vi "XuLyStringData.vi"(7 "input cluster":T3) -> (0 "error out":errorcluster, 1 "Return State":T1(ring), 2 "output cluster":T2, 3 "OUT COM 2":refnum<visa-resource-name>)   [LabVIEW 2017]
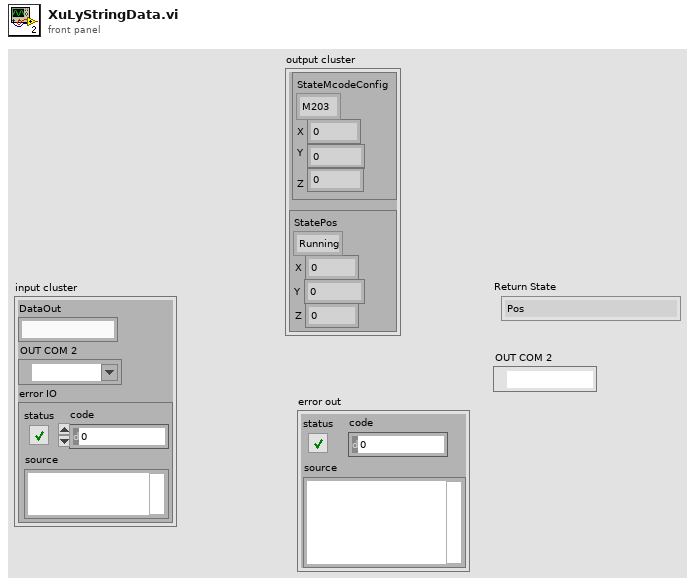
[diagram p1: front panel]
types:
  T1 = enum16{"Pos", "Config", "Echo", "OK", "Step", "Error"}
  T2 = cluster{"OUTCONFIG":cluster{"StateMcodeConfig":enum16{"M203", "M201", "M92", "M3001"}, "X":dbl, "Y":dbl, "Z":dbl}, "outPOS":cluster{"StatePos":enum16{"Running", "Waiting", "Pos", "IDLE"}, "X":dbl, "Z":dbl, "Y":dbl}}
  T3 = cluster{"DataOut":string, "OUT COM 2":refnum<visa-resource-name>, "error IO":errorcluster}
  T4 = typedef "STATE_MK4DUERETURNSTATE.ctl" = enum16{"Pos", "Config", "Echo", "OK", "Step", "Error"}
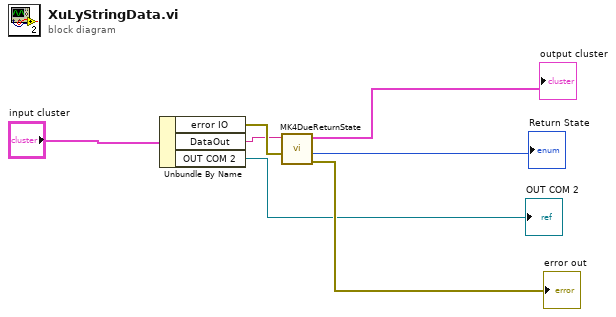
[diagram p0: block diagram]
diagram:
  n1 = Unbundle By Name("input cluster") -> ("error IO"=w5:errorcluster, "DataOut"=w4:string, "OUT COM 2"=→"OUT COM 2":refnum<visa-resource-name>)
  n2 = call "MK4DueReturnState.vi"("error IN"=w5, "String IN"=w4) -> ("error out"=→"error out":errorcluster, "Return State 2"=→"Return State":T4, "output cluster"=→"output cluster":T2)  [unwired: 4 in]
